vi "ReadUntil.vi"(0 "reference in":refnum<class "VdTcpIP.lvclass">, 1 "MatchPattern":string, 2 "timeout ms (25000)":i32=25000, 5 "Error In":errorcluster) -> (14 "reference out":refnum<class "VdTcpIP.lvclass">, 15 "Message":string, 17 "Timeout":bool, 19 "Error Out":errorcluster)   [LabVIEW 2020, in "VdTcpIP.lvclass"]
uses:
  VdTcpIP.lvclass
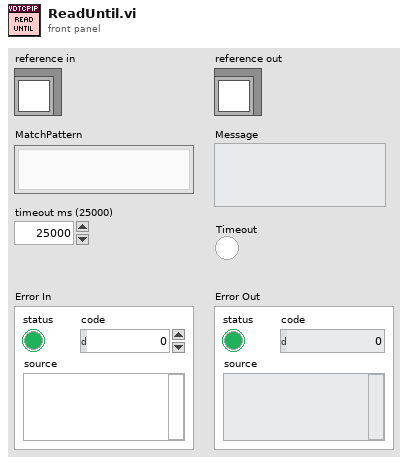
[diagram p1: front panel]
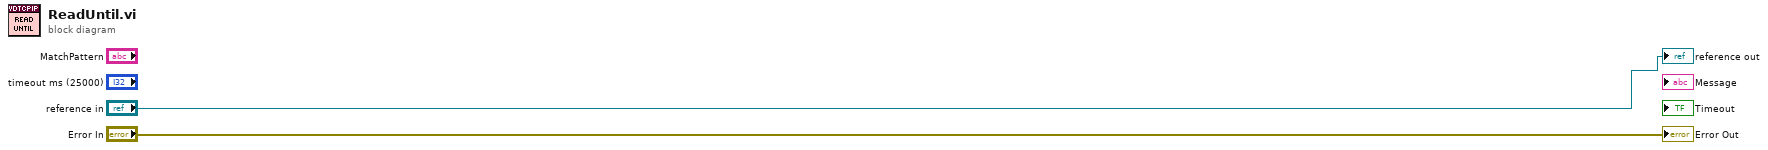
[diagram p0: block diagram]
diagram:
  "Error Out" <- "Error In"
  "reference out" <- "reference in"
